vi "test Import-Deploy-Loopback.vi"(8 "error in":errorcluster, 11 "Import-Script-Deploy.lvclass":refnum<class "Import-Script-Deploy.lvclass">) -> (0 "error out":errorcluster, 3 "Import-Script-Deploy.lvclass":refnum<class "Import-Script-Deploy.lvclass">)   [LabVIEW 2020, in "Import-Script-Deploy.lvclass"]
uses:
  Import-Script-Deploy.lvclass
  C:/Git/niveristand-custom-device-testing-tools/VeriStandTestCase/VeriStandTestCase.lvclass
  Shared/Device Parameters.ctl
  Shared/Initialization Method.ctl
  Import-Script-Deploy.lvclass/Import-Script-Deploy.ctl
  4b06c685-66bb-4135-9ad1-d89a50a95502.vi
  <vilib>/addons/_JKI Toolkits/VI Tester/TestCase.llb/TestCase.lvclass
  Import/ARINC 429 Import.lvlib
  Scripting/Ballard ARINC 429 Scripting.lvlib
  niveristand-custom-device-testing-tools/VeriStandTestUtilities/VeriStandTestUtilities.lvlib
  C:/Program Files (x86)/National Instruments/LabVIEW 2020/vi.lib/addons/_JKI Toolkits/VI Tester/TestCase.llb/TestCase.lvclass
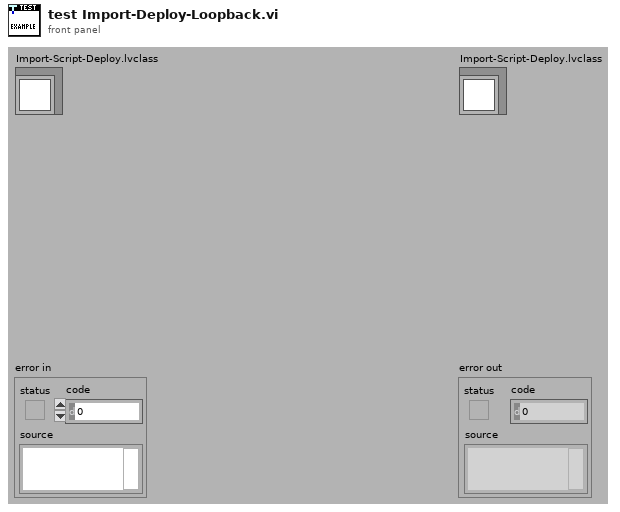
[diagram p1: front panel]
types:
  T1 = typedef "Device Parameters.ctl" = cluster{"initialization method":T2, "card number":i32, "PXI slot number":i32, "core number":i32}
  T2 = typedef "Initialization Method.ctl" = enum16{"PXI Slot Number", "Card Number"}
  T3 = typedef "VS Channels Definition for All Labels on Hardware Channel.ctl" = cluster{"hardware channel":i32, "labels":T4[]}
  T4 = typedef "VS Channels Definition for Label.ctl" = cluster{"label (Dec)":i32, "parameters":T5[], "SDI value":u8, "SDI enabled":bool, "transfer type":T9}
  T5 = typedef "VS Channel Definition for Parameter.ctl" = cluster{"name":string, "direction":T6, "default value":dbl, "unit":string, "Parameter":T7}
  T6 = typedef "Direction.ctl" = enum16{"Rx", "Tx"}
  T7 = typedef "Parameter Definition.ctl" = cluster{"start index":i32, "size":i32, "encoding":T8, "signed":bool, "scale multiplier":dbl, "scale offset":dbl}
  T8 = typedef "Encoding and Decoding.lvlib/Encoding.ctl" = enum16{"BNR", "BCD", "Discrete"}
  T9 = typedef "Transfer Type.ctl" = enum16{"Scheduled", "Acyclic", "Block", "Strobe"}
  T10 = typedef "Custom Device API.lvlib/Custom Device Item Ref.ctl" = u64
  T11 = typedef "NI_VS Workspace ExecutionAPI.lvlib/WorkspaceAPI.ctl" = refnum<k24>
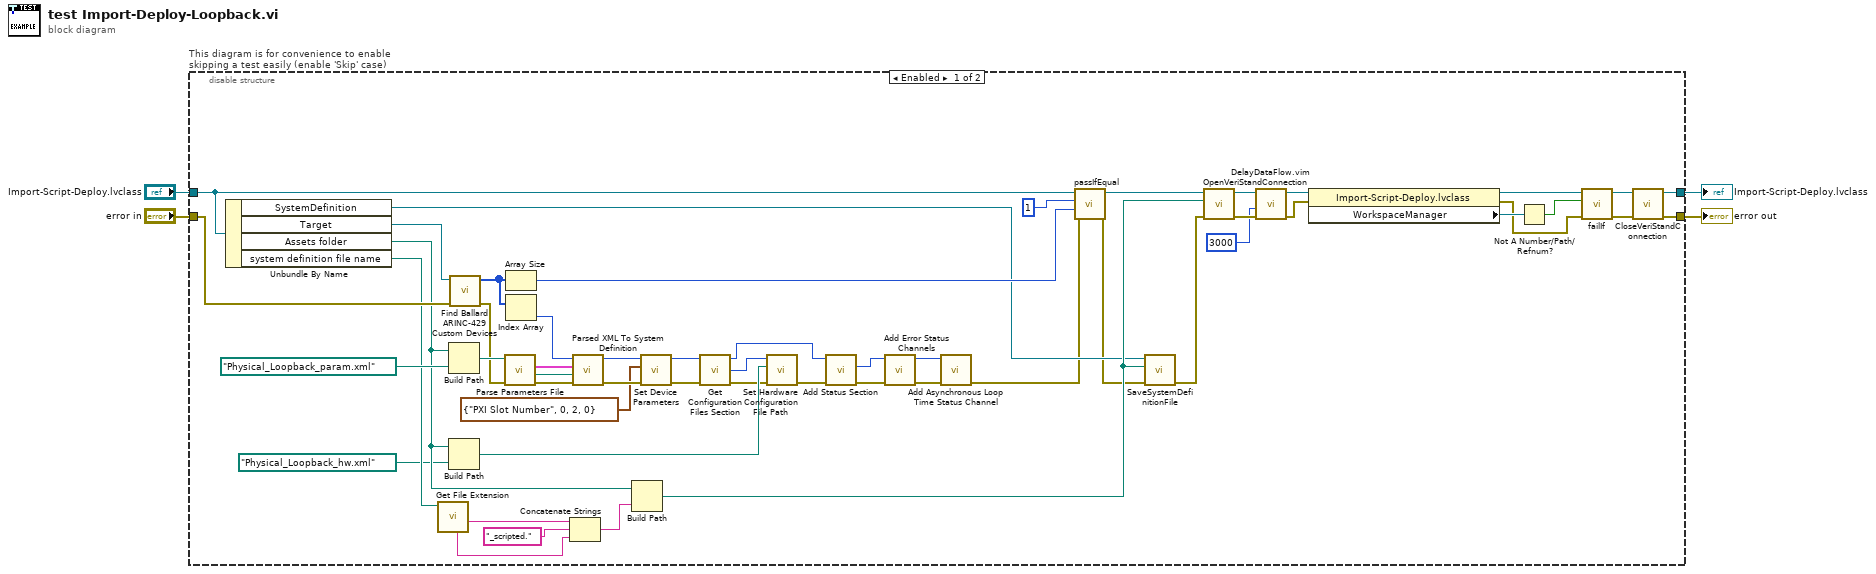
[diagram p0: block diagram]
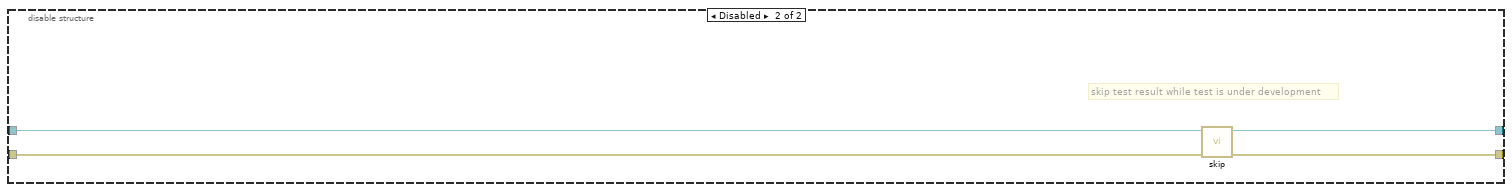
[diagram p2: hidden frame]
diagram:
  n1 = disable-structure "This diagram is for convenience to enable skipping a test easily (enable 'Skip' case)" shown="Enabled" {
    disable-tunnel: "Import-Script-Deploy.lvclass" -> [w42 w60]
    disable-tunnel: [w55 w59] -> w3
    disable-tunnel: "error in" -> [w41 w58]
    disable-tunnel: [w44 w57] -> w1
    frame Enabled {
      n2 = Unbundle By Name(w42) -> ("SystemDefinition"=w21:refnum<k24>, "Target"=w43:refnum<k24>, "Assets folder"=w18:path, "system definition file name"=w27:path)
      n3 = call <vilib>:"Get File Extension.vi"("file"=w27) -> ("filename without extension"=w26:string, "unmodified file extension"=w24:string)  [unwired: 6 in, 3 out]
      n4 = Build Path(base path=w18, name or relative path=path "Physical_Loopback_param.xml" ("Absolute or Relative Path")) -> (appended path=w48:path)
      n5 = Build Path(base path=w18, name or relative path=path "Physical_Loopback_hw.xml" ("Absolute or Relative Path")) -> (appended path=w16:path)
      n6 = call "Find Ballard ARINC-429 Custom Devices.vi"("error in"=w41, "target"=w43) -> ("error out"=w36:errorcluster, "Ballard ARINC-429 custom devices"=w40:u64[])  [unwired: 8 in]
      n7 = call "Parse Parameters File.vi"("error in"=w36, "path to XML document"=w48) -> ("error out"=w47:errorcluster, "path to XML document out"=w46:path, "ports"=w45:T3[])  [unwired: 7 in]
      n8 = Array Size(array=w40) -> (size(s)=w39:i32)
      n9 = Index Array(array=w40) -> (element=w37:u64)  [unwired: 1 in]
      n10 = Concatenate Strings(w26, "_scripted." ("string"), w24) -> (w23:string)
      n11 = call "Parsed XML To System Definition.vi"("error in"=w47, "path to XML document"=w46, "ports"=w45, "custom device ref"=w37) -> ("error out"=w30:errorcluster, "custom device ref out"=w31:T10)  [unwired: 6 in]
      n12 = Build Path(base path=w18, name or relative path=w23) -> (appended path=w22:path)
      n13 = call "Set Device Parameters.vi"("error in"=w30, "device parameters"=T1 {"initialization method"=enum."PXI Slot Number", "card number"=0, "PXI slot number"=2, "core number"=0}, "Ballard ARINC 429 custom device in"=w31) -> ("error out"=w14:errorcluster, "Ballard ARINC 429 custom device out"=w15:T10)  [unwired: 7 in]
      n14 = call "Get Configuration Files Section.vi"("error in"=w14, "Custom device Ref"=w15) -> ("error out"=w13:errorcluster, "Configuration files Ref"=w12:T10, "Custom device Ref out"=w5:T10)  [unwired: 7 in]
      n15 = call "Set Hardware Configuration File Path.vi"("error in"=w13, "Path"=w16, "Configuration files Ref"=w12) -> ("error out"=w8:errorcluster)  [unwired: 7 in, 1 out]
      n16 = call "Add Status Section.vi"("error in"=w8, "custom device ref"=w5) -> ("error out"=w7:errorcluster, "status ref"=w11:T10)  [unwired: 7 in, 1 out]
      n17 = call "Add Error Status Channels.vi"("error in"=w7, "status section ref"=w11) -> ("error out"=w10:errorcluster, "status section ref out"=w9:T10)  [unwired: 8 in]
      n18 = call "Add Asynchronous Loop Time Status Channel.vi"("error in"=w10, "status section ref"=w9) -> ("error out"=w6:errorcluster)  [unwired: 8 in, 1 out]
      n19 = call-dynamic "passIfEqual.vi"("error in (no error)"=w6, "y"=w39, "x"=1 ("size(s)"), "TestCase in"=w42) -> ("error out"=w19:errorcluster, "TestCase out"=w35:refnum<class "Import-Script-Deploy.lvclass">)  [unwired: 6 in]
      n20 = call "SaveSystemDefinitionFile.vi"("error in (no error)"=w19, "System Definition File in"=w22, "System Definition Reference in"=w21) -> ("error out"=w20:errorcluster)  [unwired: 7 in, 1 out]
      n21 = call-dynamic "OpenVeriStandConnection.vi"("error in (no error)"=w20, "System Definition File"=w22, "VeriStand Test Case in"=w35) -> ("error out"=w34:errorcluster, "VeriStand Test Case out"=w33:refnum<class "Import-Script-Deploy.lvclass">)  [unwired: 6 in, 1 out]
      n22 = call "DelayDataFlow.vim"("value in"=w34, "milliseconds to wait"=u32 3000) -> ("value out"=w56:errorcluster)  [unwired: 2 in, 1 out]
      n23 = property class="Import-Script-Deploy.lvclass"(reference=w33, error in=w56) -> (reference out=w54:refnum<class "Import-Script-Deploy.lvclass">, error out=w49:errorcluster, "WorkspaceManager"=w51:T11)
      n24 = Not A Number/Path/Refnum?(number/path/refnum=w51) -> (NaN/Path/Refnum?=w50:bool)
      n25 = call-dynamic "failIf.vi"("error in (no error)"=w49, "fail"=w50, "TestCase in"=w54) -> ("error out"=w52:errorcluster, "TestCase out"=w53:refnum<class "Import-Script-Deploy.lvclass">)  [unwired: 7 in]
      n26 = call-dynamic "CloseVeriStandConnection.vi"("error in (no error)"=w52, "VeriStand Test Case in"=w53) -> ("error out"=w55:errorcluster, "VeriStand Test Case out"=w44:refnum<class "Import-Script-Deploy.lvclass">)  [unwired: 8 in]
    }
    frame Disabled {
      # "skip test result while test is under development"
      n27 = call <vilib>:"skip.vi"("error in (no error)"=w58, "TestCase in"=w60) -> ("error out"=w59:errorcluster, "TestCase out"=w57:refnum<class "Import-Script-Deploy.lvclass">)  [unwired: 8 in]
    }
  }
  "error out" <- w3
  "Import-Script-Deploy.lvclass" <- w1
